vi "Begin.vi"(8 "error in":errorcluster) -> (0 "error out":errorcluster)   [LabVIEW 2014]
doc: "Called before other user functions, this VI is expected to open initial I/O refnums, load in file data, and do all program initialization. Notice that the <B>error out</B> terminal is simply used for data flow. Wiring it to other structures or subVIs ensures that this VI runs first."
uses:
  <vilib>/Rock Robotics/WPI/DriverStation/WPI_DriverStationRobotMode2.ctl
  <vilib>/Rock Robotics/SystemInterfaces/DIO/FPGA_DIOPWMChannel.ctl
  <vilib>/Rock Robotics/WPI/Joystick/WPI_JoystickDeviceEnum.ctl
  <vilib>/Rock Robotics/WPI/Solenoid/WPI_SolenoidChannel.ctl
  <vilib>/Rock Robotics/WPI/SafetyOutput/WPI_SafetyOutputConfigMenu.ctl
  <vilib>/Rock Robotics/SystemInterfaces/DIO/FPGA_DIOChannel.ctl
  <vilib>/Rock Robotics/SystemInterfaces/AI/FPGA_AIChannel.ctl
  <vilib>/Rock Robotics/WPI/Encoder/WPI_EncoderType.ctl
  Robot Global Data.vi
  <vilib>/Rock Robotics/WPI/MotorControl/WPI_MotorControlOpen Victor.vi
  <vilib>/Rock Robotics/WPI/Solenoid/WPI_SolenoidOpenDouble.vi
  <vilib>/Rock Robotics/WPI/Switch/WPI_SwitchOpenLimit.vi
  <vilib>/Rock Robotics/WPI/Counter/WPI_CounterDigitalInputToDigitalSource.vi
  <vilib>/Rock Robotics/WPI/RobotDrive/WPI_RobotDriveOpen2MotorWithTalon.vi
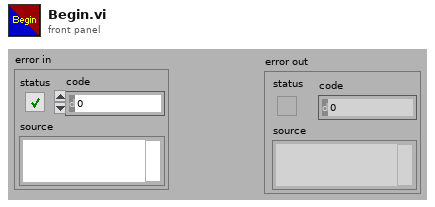
[diagram p1: front panel]
types:
  T1 = typedef "WPI_EncoderType.ctl" = enum16{"1x", "2x", "4x"}
  T2 = typedef "FPGA_AIChannel.ctl" = enum8{"AI 0", "AI 1", "AI 2", "AI 3", "AI MXP 0", "AI MXP 1", "AI MXP 2", "AI MXP 3", "Invalid"}
  T3 = typedef "FPGA_DIOChannel.ctl" = enum8{"DIO 0", "DIO 1", "DIO 2", "DIO 3", "DIO 4", "DIO 5", "DIO 6", "DIO 7", "DIO 8", "DIO 9", "DIO MXP 0", "DIO MXP 1", "DIO MXP 2", "DIO MXP 3", "DIO MXP 4", "DIO MXP 5", "DIO MXP 6", "DIO MXP 7", "DIO MXP 8", "DIO MXP 9", "DIO MXP 10", "DIO MXP 11", "DIO MXP 12", "DIO MXP 13", "DIO MXP 14", "DIO MXP 15", "Invalid"}
  T4 = typedef "WPI_SafetyOutputConfigMenu.ctl" = enum16{"Enable", "Disable"}
  T5 = typedef "WPI_SolenoidChannel.ctl" = enum8{"Solenoid 0", "Solenoid 1", "Solenoid 2", "Solenoid 3", "Solenoid 4", "Solenoid 5", "Solenoid 6", "Solenoid 7", "Invalid"}
  T6 = typedef "FPGA_DIOPWMChannel.ctl" = enum8{"PWM 0", "PWM 1", "PWM 2", "PWM 3", "PWM 4", "PWM 5", "PWM 6", "PWM 7", "PWM 8", "PWM 9", "PWM MXP 0", "PWM MXP 1", "PWM MXP 2", "PWM MXP 3", "PWM MXP 4", "PWM MXP 5", "PWM MXP 6", "PWM MXP 7", "PWM MXP 8", "PWM MXP 9", "Invalid"}
  T7 = typedef "WPI_JoystickDeviceEnum.ctl" = enum16{"USB 0", "USB 1", "USB 2", "USB 3", "USB 4", "USB 5"}
  T8 = typedef "WPI_DriverStationRobotMode2.ctl" = enum16{"Autonomous Disabled", "Autonomous Enabled", "Teleop Disabled", "Teleop Enabled", "Disconnected", "Finish", "Test Disabled", "Test Enabled", "Emergency Stopped"}
  T9 = typedef "WPI_RobotDriveDevRef.ctl" = cluster{"DevStatus":errorcluster, "Motors[]":T10[], "Square Inputs":bool, "Max Output":dbl}
  T10 = typedef "WPI_MotorControlDeviceRef.ctl" = cluster{"DeviceStatus":errorcluster, "Type":T11, "PWM":cluster{"Controller":T12, "PWM Channel":T6, "DeadBand":T13}, "CAN":cluster{"Device Number":u8, "Control Mode":T14, "Semaphore":T15, "Max Vout":dbl, "TalonSRX Control Mode":T16}, "Invert":bool, "TransformRef":T17, "InvTransformRef":T17}
  T11 = typedef "WPI_MotorControlType.ctl" = enum16{"PWM", "CAN", "CANTalonSRX"}
  T12 = typedef "FPGA_TypedefDigitalModule.ctl" = enum16{"Controller 1"}
  T13 = typedef "WPI_PWMDeadband.ctl" = cluster{"Name":string, "maxPositivePwm":i32, "minPositivePwm":i32, "centerPwm":i32, "maxNegativePwm":i32, "minNegativePwm":i32, "angularRange":u16}
  T14 = typedef "WPI_CANJaguar_ControlMode.ctl" = enum8{"Percent VBus", "Current", "Speed", "Position", "Voltage"}
  T15 = typedef "Semaphore RefNum" = refnum<k1>
  T16 = typedef "WPI_CANTalonSRX_APIControlMode.ctl" = enum8{"Percent VBus", "Speed", "Position", "Slave", "Unchanged / Invalid"}
  T17 = typedef "WPI_PWMTransform_ConPane.ctl" = refnum<vi>
  T18 = typedef "WPI_JoystickDevRef.ctl" = cluster{"Device":T7}
  T19 = typedef "WPI_SolenoidDevRef.ctl" = cluster{"DevStatus":errorcluster, "Pneumatics Control Module":u8, "Forward Solenoid Channel":T5, "Reverse Solenoid Channel":T5}
  T20 = typedef "WPI_AnalogChannelDevRef.ctl" = cluster{"DevStatus":errorcluster, "Controller":T21, "Analog Channel":T2}
  T21 = typedef "FPGA_TypedefAnalogModule.ctl" = enum16{"Controller 1"}
  T22 = typedef "WPI_DigitalInputDevRef.ctl" = cluster{"DevStatus":errorcluster, "DIO Channel":T3, "Controller":T12}
  T23 = typedef "WPI_SwitchDevRef.ctl" = cluster{"DevStatus":errorcluster, "DIO Channel":T3, "Controller":T12, "CntIndex":T24, "Normally Closed":bool}
  T24 = typedef "FPGA_CounterCtrSystemIndex.ctl" = enum8{"Ctr 0", "Ctr 1", "Ctr 2", "Ctr 3", "Ctr 4", "Ctr 5", "Ctr 6", "Ctr 7", "Invalid"}
  T25 = typedef "FPGA_CounterEncoderSourceConvertionLVSourceType.ctl" = cluster{"DevStatus":errorcluster, "AnalogTriggerMode?":bool, "DigitalMode":cluster{"Controller":T12, "DIO Channel":T26}, "AnalogTriggerMode":cluster{"AnalogTriggerIndex":T27, "OutputType":T28}}
  T26 = typedef "FPGA_DIODigitalSourceChannel.ctl" = enum8{"DIO 0", "DIO 1", "DIO 2", "DIO 3", "DIO 4", "DIO 5", "DIO 6", "DIO 7", "DIO 8", "DIO 9", "DIO MXP 0", "DIO MXP 1", "DIO MXP 2", "DIO MXP 3", "DIO MXP 4", "DIO MXP 5", "DIO MXP 6", "DIO MXP 7", "DIO MXP 8", "DIO MXP 9", "DIO MXP 10", "DIO MXP 11", "DIO MXP 12", "DIO MXP 13", "DIO MXP 14", "DIO MXP 15", "Disabled"}
  T27 = typedef "FPGA_AnalogTriggerIndex.ctl" = enum8{"Trig 0", "Trig 1", "Trig 2", "Trig 3", "Trig 4", "Trig 5", "Trig 6", "Trig 7", "Invalid"}
  T28 = typedef "FPGA_AnalogTriggerOutType.ctl" = enum16{"InWindow", "TriggerState", "Rising", "Falling"}
  T29 = typedef "WPI_EncoderDevRef.ctl" = cluster{"DevStatus":errorcluster, "EncoderIndex":T30, "CounterIndex":T24, "DistancePerCount":dbl, "Decoding Type":T1}
  T30 = typedef "FPGA_EncoderIdx.ctl" = enum8{"Enc 0", "Enc 1", "Enc 2", "Enc 3", "Enc 4", "Enc 5", "Enc 6", "Enc 7", "Invalid"}
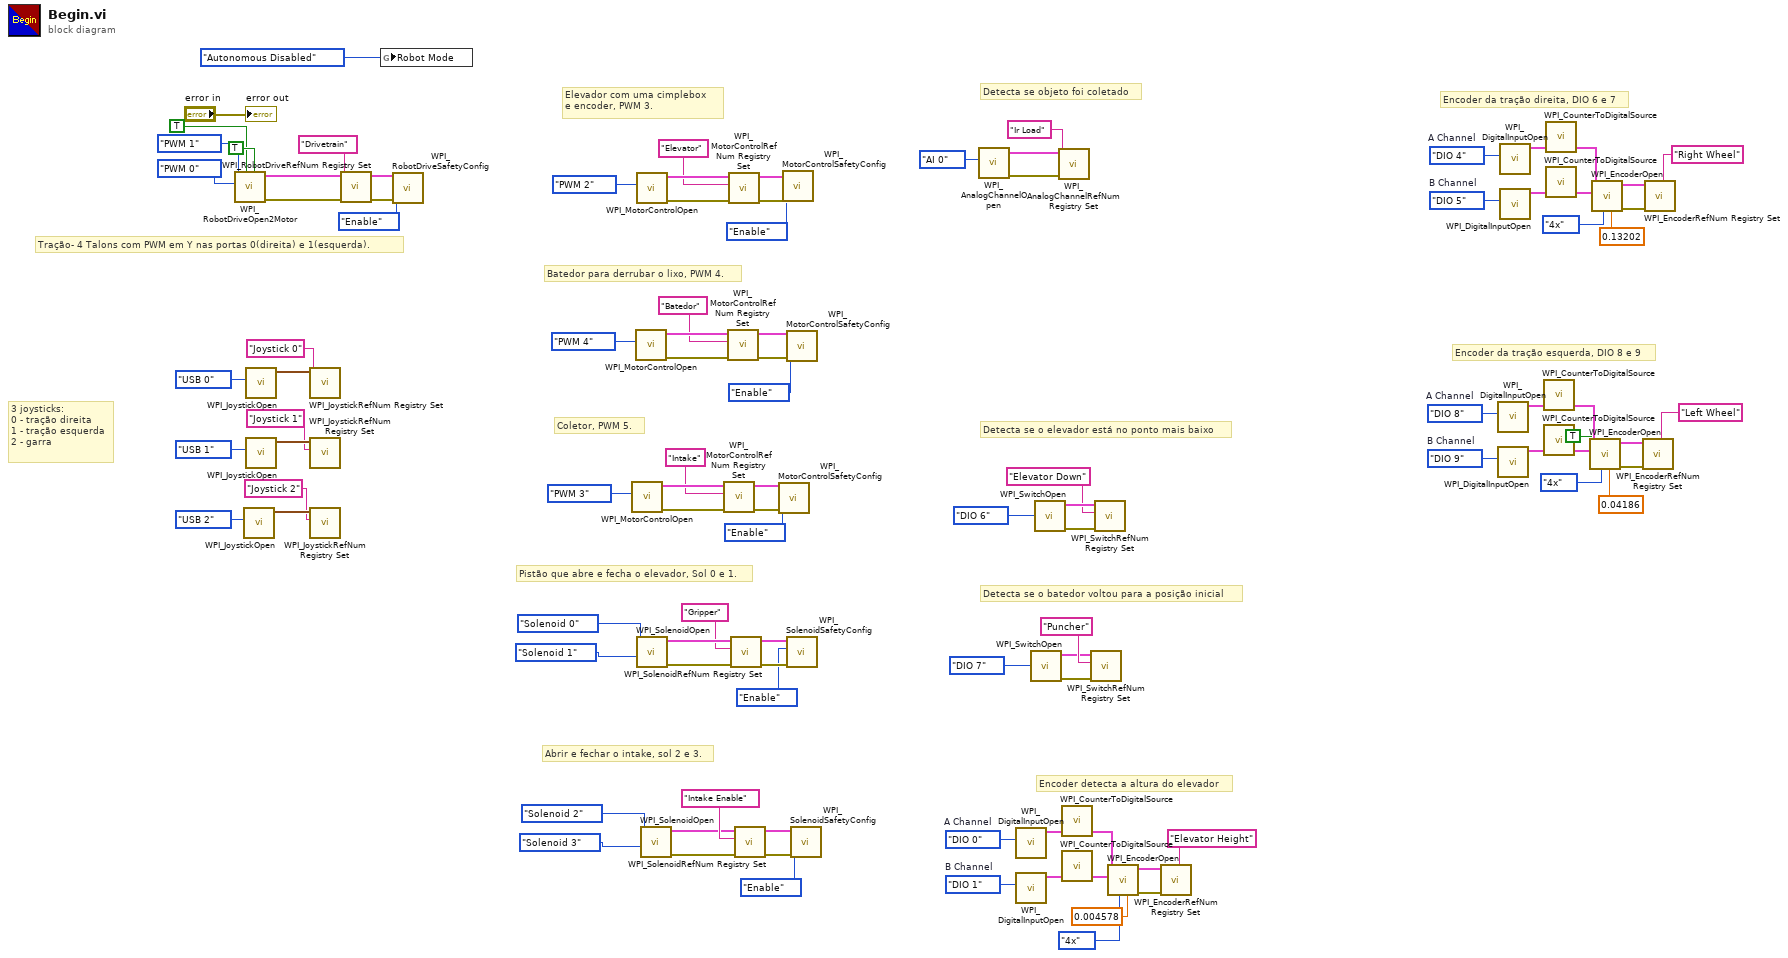
[diagram p0: block diagram]
diagram:
  w20 = FPGA_DIOChannel."DIO 9"  # B Channel
  w19 = FPGA_DIOChannel."DIO 8"  # A Channel
  w21 = FPGA_DIOChannel."DIO 5"  # B Channel
  w22 = FPGA_DIOChannel."DIO 4"  # A Channel
  w40 = FPGA_DIOChannel."DIO 1"  # B Channel
  w39 = FPGA_DIOChannel."DIO 0"  # A Channel
  # "Encoder da tração esquerda, DIO 8 e 9"
  # "Encoder da tração direita, DIO 6 e 7"
  # "Encoder detecta a altura do elevador"
  # "Detecta se o batedor voltou para a posição inicial"
  # "Detecta se o elevador está no ponto mais baixo"
  # "Detecta se objeto foi coletado"
  # "Abrir e fechar o intake, sol 2 e 3."
  # "Pistão que abre e fecha o elevador, Sol 0 e 1."
  # "Coletor, PWM 5."
  # "Batedor para derrubar o lixo, PWM 4."
  # "Elevador com uma cimplebox\ne encoder, PWM 3."
  # "3 joysticks:\n0 - tração direita\n1 - tração esquerda\n2 - garra"
  # "Tração- 4 Talons com PWM em Y nas portas 0(direita) e 1(esquerda)."
  n1 = call-poly <vilib>:"WPI_RobotDriveOpen2Motor.vi"("Right Motor Inverted"=TRUE, "Left Motor Inverted"=TRUE, "Right Motor"=FPGA_DIOPWMChannel."PWM 0", "Left Motor"=FPGA_DIOPWMChannel."PWM 1") -> ("error out"=w101:errorcluster, "RobotDriveDevRef"=w102:T9)  [unwired: 6 in]
  n2 = call <vilib>:"WPI_JoystickOpen.vi"("JoystickDevice"=WPI_JoystickDeviceEnum."USB 2") -> ("JoystickDevRef"=w92:T18)  [unwired: 10 in]
  n3 = call <vilib>:"WPI_JoystickOpen.vi"("JoystickDevice"=WPI_JoystickDeviceEnum."USB 0") -> ("JoystickDevRef"=w97:T18)  [unwired: 10 in]
  n4 = call <vilib>:"WPI_JoystickOpen.vi"("JoystickDevice"=WPI_JoystickDeviceEnum."USB 1") -> ("JoystickDevRef"=w94:T18)  [unwired: 10 in]
  n5 = call <vilib>:"WPI_JoystickRefNum Registry Set.vi"("refnum name"="Joystick 0", "JoystickDevRef"=w97) -> ()  [unwired: 8 in, 2 out]
  n6 = call <vilib>:"WPI_JoystickRefNum Registry Set.vi"("refnum name"="Joystick 1", "JoystickDevRef"=w94) -> ()  [unwired: 8 in, 2 out]
  n7 = call <vilib>:"WPI_JoystickRefNum Registry Set.vi"("refnum name"="Joystick 2", "JoystickDevRef"=w92) -> ()  [unwired: 8 in, 2 out]
  n8 = call <vilib>:"WPI_RobotDriveRefNum Registry Set.vi"("error in (no error)"=w101, "refnum name"="Drivetrain", "RobotDriveDevRef"=w102) -> ("error out"=w72:errorcluster, "RobotDriveDevRef"=w71:T9)  [unwired: 7 in]
  n9 = global write "Robot Global Data.vi" "Robot Mode"(WPI_DriverStationRobotMode2."Autonomous Disabled" ("Robot Mode")) -> ()
  n10 = call <vilib>:"WPI_RobotDriveSafetyConfig.vi"("error in (no error)"=w72, "mode"=WPI_SafetyOutputConfigMenu."Enable", "RobotDriveDevRef"=w71) -> ()  [unwired: 7 in, 2 out]
  n11 = call-poly <vilib>:"WPI_MotorControlOpen.vi"("PWM Channel"=FPGA_DIOPWMChannel."PWM 3") -> ("error out"=w79:errorcluster, "MotorControlDeviceRef"=w80:T10)  [unwired: 9 in]
  n12 = call-poly <vilib>:"WPI_MotorControlOpen.vi"("PWM Channel"=FPGA_DIOPWMChannel."PWM 4") -> ("error out"=w83:errorcluster, "MotorControlDeviceRef"=w84:T10)  [unwired: 9 in]
  n13 = call-poly <vilib>:"WPI_MotorControlOpen.vi"("PWM Channel"=FPGA_DIOPWMChannel."PWM 2") -> ("error out"=w87:errorcluster, "MotorControlDeviceRef"=w88:T10)  [unwired: 9 in]
  n14 = call-poly <vilib>:"WPI_SolenoidOpen.vi"("Reverse Solenoid Channel"=WPI_SolenoidChannel."Solenoid 1", "Forward Solenoid Channel"=WPI_SolenoidChannel."Solenoid 0" ("Solenoid Channel")) -> ("error out"=w75:errorcluster, "SolenoidDevRef"=w76:T19)  [unwired: 8 in]
  n15 = call-poly <vilib>:"WPI_SolenoidOpen.vi"("Reverse Solenoid Channel"=WPI_SolenoidChannel."Solenoid 3", "Forward Solenoid Channel"=WPI_SolenoidChannel."Solenoid 2" ("Solenoid Channel")) -> ("error out"=w50:errorcluster, "SolenoidDevRef"=w49:T19)  [unwired: 8 in]
  n16 = call <vilib>:"WPI_MotorControlRefNum Registry Set.vi"("error in (no error)"=w79, "refnum name"="Intake", "MotorControlDevRef"=w80) -> ("error out"=w63:errorcluster, "MotorControlDevRef"=w62:T10)  [unwired: 7 in]
  n17 = call <vilib>:"WPI_MotorControlRefNum Registry Set.vi"("error in (no error)"=w83, "refnum name"="Batedor", "MotorControlDevRef"=w84) -> ("error out"=w66:errorcluster, "MotorControlDevRef"=w65:T10)  [unwired: 7 in]
  n18 = call <vilib>:"WPI_MotorControlRefNum Registry Set.vi"("error in (no error)"=w87, "refnum name"="Elevator", "MotorControlDevRef"=w88) -> ("error out"=w69:errorcluster, "MotorControlDevRef"=w68:T10)  [unwired: 7 in]
  n19 = call <vilib>:"WPI_SolenoidRefNum Registry Set.vi"("error in (no error)"=w75, "refnum name"="Gripper", "SolenoidDevRef"=w76) -> ("error out"=w59:errorcluster, "SolenoidDevRef"=w58:T19)  [unwired: 7 in]
  n20 = call <vilib>:"WPI_SolenoidRefNum Registry Set.vi"("error in (no error)"=w50, "refnum name"="Intake Enable", "SolenoidDevRef"=w49) -> ("error out"=w54:errorcluster, "SolenoidDevRef"=w55:T19)  [unwired: 7 in]
  n21 = call <vilib>:"WPI_MotorControlSafetyConfig.vi"("error in (no error)"=w63, "mode"=WPI_SafetyOutputConfigMenu."Enable", "MotorControlDevRef"=w62) -> ()  [unwired: 7 in, 2 out]
  n22 = call <vilib>:"WPI_MotorControlSafetyConfig.vi"("error in (no error)"=w69, "mode"=WPI_SafetyOutputConfigMenu."Enable", "MotorControlDevRef"=w68) -> ()  [unwired: 7 in, 2 out]
  n23 = call <vilib>:"WPI_MotorControlSafetyConfig.vi"("error in (no error)"=w66, "mode"=WPI_SafetyOutputConfigMenu."Enable", "MotorControlDevRef"=w65) -> ()  [unwired: 7 in, 2 out]
  n24 = call <vilib>:"WPI_SolenoidSafetyConfig.vi"("error in (no error)"=w59, "mode"=WPI_SafetyOutputConfigMenu."Enable", "SolenoidDevRef"=w58) -> ()  [unwired: 7 in, 2 out]
  n25 = call <vilib>:"WPI_SolenoidSafetyConfig.vi"("error in (no error)"=w54, "mode"=WPI_SafetyOutputConfigMenu."Enable", "SolenoidDevRef"=w55) -> ()  [unwired: 7 in, 2 out]
  n26 = call <vilib>:"WPI_AnalogChannelOpen.vi"("Analog Channel"=FPGA_AIChannel."AI 0") -> ("error out"=w9:errorcluster, "AIDeviceRef"=w10:T20)  [unwired: 9 in]
  n27 = call <vilib>:"WPI_DigitalInputOpen.vi"("DIO Channel"=w39) -> ("DigitalInputDevRef"=w36:T22)  [unwired: 2 in, 8 out]
  n28 = call <vilib>:"WPI_DigitalInputOpen.vi"("DIO Channel"=w40) -> ("DigitalInputDevRef"=w37:T22)  [unwired: 2 in, 8 out]
  n29 = call-poly <vilib>:"WPI_SwitchOpen.vi"("DIO Channel"=FPGA_DIOChannel."DIO 7") -> ("error out"=w42:errorcluster, "SwitchDevRef"=w43:T23)  [unwired: 9 in]
  n30 = call-poly <vilib>:"WPI_SwitchOpen.vi"("DIO Channel"=FPGA_DIOChannel."DIO 6") -> ("error out"=w47:errorcluster, "SwitchDevRef"=w46:T23)  [unwired: 9 in]
  n31 = call <vilib>:"WPI_AnalogChannelRefNum Registry Set.vi"("error in (no error)"=w9, "refnum name"="Ir Load", "AIDeviceRef"=w10) -> ()  [unwired: 7 in, 2 out]
  n32 = call-poly <vilib>:"WPI_CounterToDigitalSource.vi"("DigitalInputDevRef"=w36) -> ("Digital Source"=w35:T25)  [unwired: 6 out]
  n33 = call-poly <vilib>:"WPI_CounterToDigitalSource.vi"("DigitalInputDevRef"=w37) -> ("Digital Source"=w38:T25)  [unwired: 6 out]
  n34 = call <vilib>:"WPI_SwitchRefNum Registry Set.vi"("error in (no error)"=w42, "refnum name"="Puncher", "SwitchDevRef"=w43) -> ()  [unwired: 7 in, 2 out]
  n35 = call <vilib>:"WPI_SwitchRefNum Registry Set.vi"("error in (no error)"=w47, "refnum name"="Elevator Down", "SwitchDevRef"=w46) -> ()  [unwired: 7 in, 2 out]
  n36 = call <vilib>:"WPI_EncoderOpen.vi"("DistancePerCount"=0.004578, "Decoding Type"=WPI_EncoderType."4x", "BSource"=w38, "ASource"=w35) -> ("error out"=w33:errorcluster, "EncoderDevRef"=w32:T29)  [unwired: 4 in, 2 out]
  n37 = call <vilib>:"WPI_EncoderRefNum Registry Set.vi"("error in (no error)"=w33, "refnum name"="Elevator Height", "EncoderDevRef"=w32) -> ()  [unwired: 7 in, 2 out]
  n38 = call <vilib>:"WPI_DigitalInputOpen.vi"("DIO Channel"=w19) -> ("DigitalInputDevRef"=w16:T22)  [unwired: 2 in, 8 out]
  n39 = call <vilib>:"WPI_DigitalInputOpen.vi"("DIO Channel"=w20) -> ("DigitalInputDevRef"=w17:T22)  [unwired: 2 in, 8 out]
  n40 = call <vilib>:"WPI_DigitalInputOpen.vi"("DIO Channel"=w22) -> ("DigitalInputDevRef"=w25:T22)  [unwired: 2 in, 8 out]
  n41 = call <vilib>:"WPI_DigitalInputOpen.vi"("DIO Channel"=w21) -> ("DigitalInputDevRef"=w24:T22)  [unwired: 2 in, 8 out]
  n42 = call-poly <vilib>:"WPI_CounterToDigitalSource.vi"("DigitalInputDevRef"=w16) -> ("Digital Source"=w15:T25)  [unwired: 6 out]
  n43 = call-poly <vilib>:"WPI_CounterToDigitalSource.vi"("DigitalInputDevRef"=w17) -> ("Digital Source"=w18:T25)  [unwired: 6 out]
  n44 = call-poly <vilib>:"WPI_CounterToDigitalSource.vi"("DigitalInputDevRef"=w25) -> ("Digital Source"=w26:T25)  [unwired: 6 out]
  n45 = call-poly <vilib>:"WPI_CounterToDigitalSource.vi"("DigitalInputDevRef"=w24) -> ("Digital Source"=w23:T25)  [unwired: 6 out]
  n46 = call <vilib>:"WPI_EncoderOpen.vi"("DistancePerCount"=0.04186, "Decoding Type"=WPI_EncoderType."4x", "Invert Direction (False)"=TRUE, "BSource"=w18, "ASource"=w15) -> ("error out"=w13:errorcluster, "EncoderDevRef"=w12:T29)  [unwired: 3 in, 2 out]
  n47 = call <vilib>:"WPI_EncoderOpen.vi"("DistancePerCount"=0.13202, "Decoding Type"=WPI_EncoderType."4x", "BSource"=w23, "ASource"=w26) -> ("error out"=w28:errorcluster, "EncoderDevRef"=w29:T29)  [unwired: 4 in, 2 out]
  n48 = call <vilib>:"WPI_EncoderRefNum Registry Set.vi"("error in (no error)"=w13, "refnum name"="Left Wheel", "EncoderDevRef"=w12) -> ()  [unwired: 7 in, 2 out]
  n49 = call <vilib>:"WPI_EncoderRefNum Registry Set.vi"("error in (no error)"=w28, "refnum name"="Right Wheel", "EncoderDevRef"=w29) -> ()  [unwired: 7 in, 2 out]
  "error out" <- "error in"
